vi "read_params.vi"(8 "error in (no error)":errorcluster, 11 "BayesianGaussianMixture in":refnum<class "BayesianGaussianMixture.lvclass">) -> (0 "error out":errorcluster, 2 "params":T1={"n_components"=1.0, "covariance_type"="full", "tol"=0.001, "reg_covar"=1e-06, "max_iter"=100.0, "n_init"=1.0, "init_params"="kmeans", "weight_concentration_prior_type"="dirichlet_process", "weight_concentration_prior"={"weight_concentration_prior_type"="None", "weight_concentration_prior_float"=0.0}, "mean_precision_prior"=0.9999999999999, "mean_prior"={"mean_prior_type"="None", "mean_prior_list"=[]}, "degrees_of_freedom_prior"={"degrees_of_freedom_prior_type"="None", "degrees_of_freedom_prior_float"=0.0}, "covariance_prior"={"covariance_prior_type"="None", "covariance_prior_float"=0.0, "covariance_prior_list"=[]}, "random_state"=0.0, "warm_start"=FALSE, "verbose"=0.0, "verbose_interval"=10.0}, 3 "BayesianGaussianMixture out":refnum<class "BayesianGaussianMixture.lvclass">)   [LabVIEW 2020, in "BayesianGaussianMixture.lvclass"]
uses:
  BayesianGaussianMixture.lvclass
  Controls/bayesian_gaussian_mixture_params.ctl
  BayesianGaussianMixture.lvclass/BayesianGaussianMixture.ctl
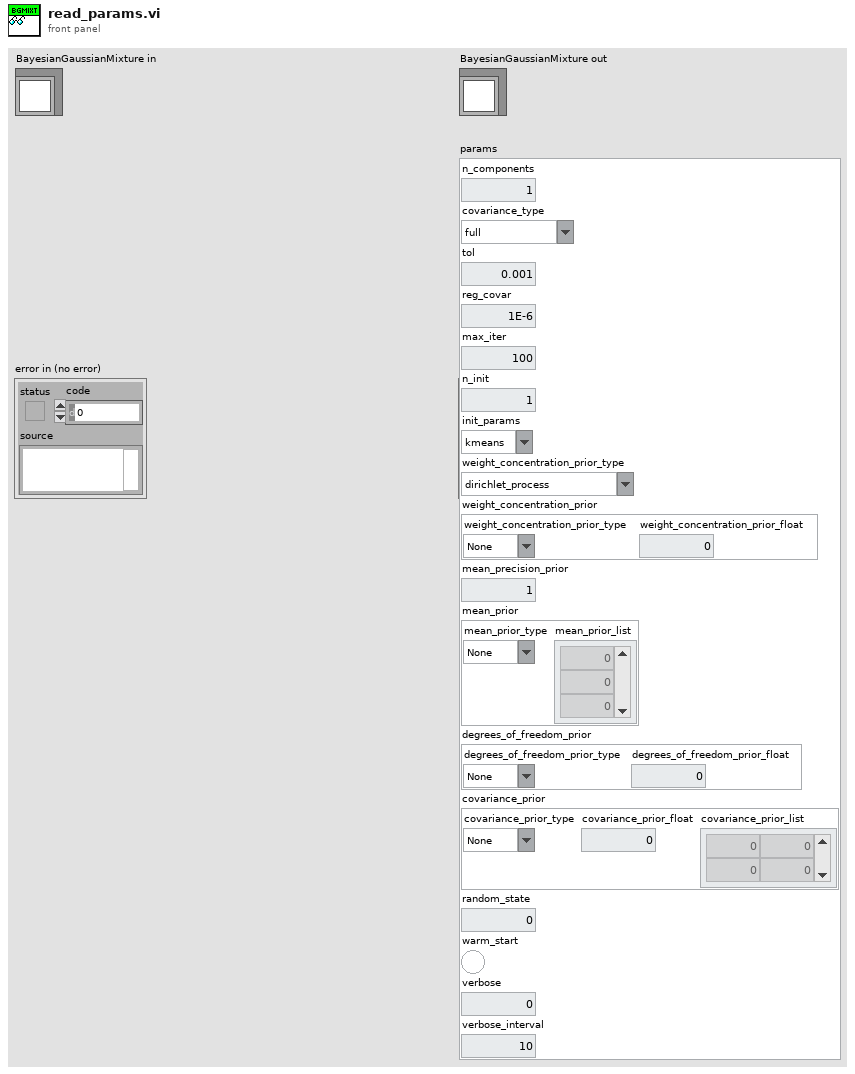
[diagram p1: front panel]
types:
  T1 = typedef "bayesian_gaussian_mixture_params.ctl" = cluster{"n_components":dbl, "covariance_type":string, "tol":dbl, "reg_covar":dbl, "max_iter":dbl, "n_init":dbl, "init_params":string, "weight_concentration_prior_type":string, "weight_concentration_prior":cluster{"weight_concentration_prior_type":string, "weight_concentration_prior_float":dbl}, "mean_precision_prior":dbl, "mean_prior":cluster{"mean_prior_type":string, "mean_prior_list":dbl[]}, "degrees_of_freedom_prior":cluster{"degrees_of_freedom_prior_type":string, "degrees_of_freedom_prior_float":dbl}, "covariance_prior":cluster{"covariance_prior_type":string, "covariance_prior_float":dbl, "covariance_prior_list":dbl[][]}, "random_state":dbl, "warm_start":bool, "verbose":dbl, "verbose_interval":dbl}
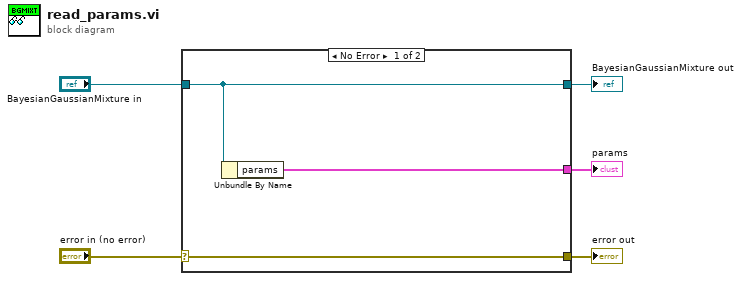
[diagram p0: block diagram]
diagram:
  n1 = case shown="No Error" "error in (no error)" {
    selector: "error in (no error)" -> [w8 w9]
    tunnel: [w8 w9] -> w4
    tunnel: [w7 w10] -> w2
    tunnel: "BayesianGaussianMixture in" -> [w7 w10]
    tunnel: [w6 _] -> w1
    frame No Error {
      n2 = Unbundle By Name(w7) -> ("params"=w6:T1)
    }
    frame Error {
    }
  }
  "error out" <- w4
  "BayesianGaussianMixture out" <- w2
  "params" <- w1
